vi "Add Custom Device to Sys Def.vi"(9 "Test Number":string="1", 10 "Custom Device Configuration File Path":path=path "C:/Users/admin/Desktop/Custom Device Tests/VeriStandProject/Custom Device Configurations/instrument_addon_udp_config.dat", 11 "nivssdfFile":string="C:\\Users\\admin\\Desktop\\Custom Device Tests\\VeriStandProject\\Instrument Custom Device Test.nivssdf") -> (0 "error out":errorcluster={"status"=TRUE, "code"=1430, "source"="Open/Create/Replace Datalog in Instrument System Definition API.lvlibp:Advanced System Definition.lvlib:Sysdef.LoadFile.vi->Instrument System Definition API.lvlibp:ImportExport.lvlib:File Interface.lvclass:Read File.vi->Instrument System Definition API.lvlibp:ImportExport.lvlib:Import Custom Device Configuration.vi->Instrument System Definition API.lvlibp:Create Instrument Custom Device.vi->Add Custom Device to Sys Def.vi<APPEND>\ninstrument_addon_udp_config.dat"}, 1 "SysDef Save error":string, 3 "Test Sys Def Path":string)   [LabVIEW 2015]
uses:
  Instrument System Definition API.lvlibp
  NationalInstruments.VeriStand.SystemDefinitionAPI
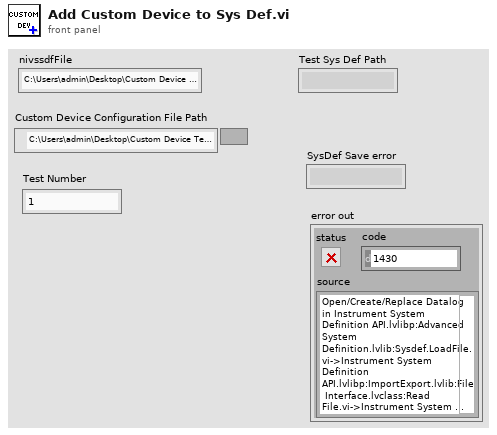
[diagram p1: front panel]
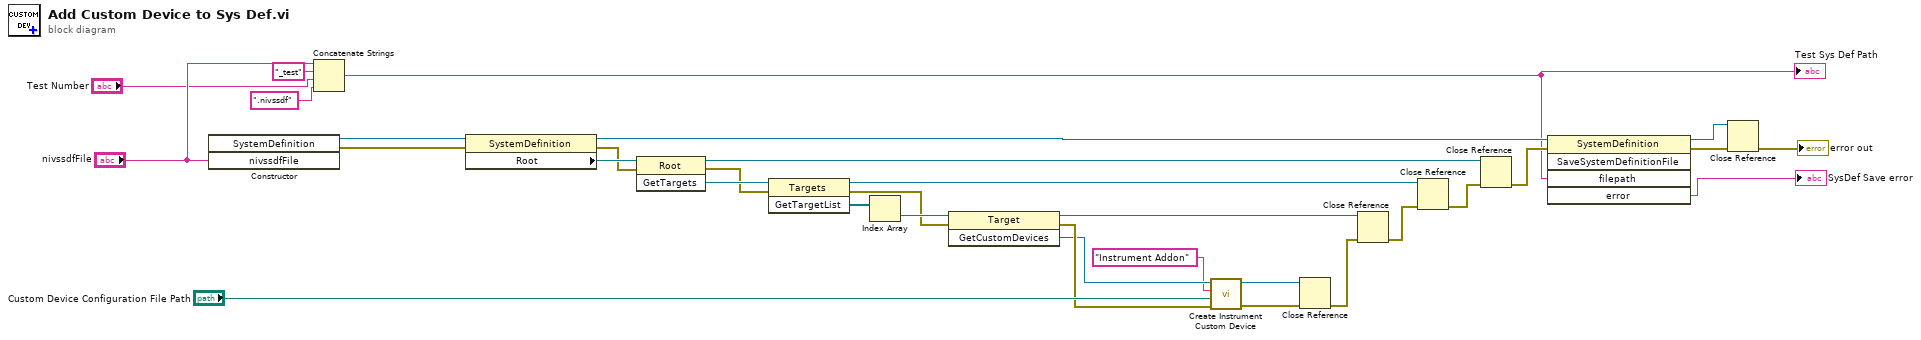
[diagram p0: block diagram]
diagram:
  n1 = constructor class="SystemDefinition"("nivssdfFile"="nivssdfFile") -> (reference out=w7:refnum<k24>, error out=w31:errorcluster)  [unwired: 3 in, 2 out]
  n2 = Concatenate Strings("nivssdfFile", "_test" ("string"), "Test Number", ".nivssdf" ("string")) -> (w3:string)
  "Test Sys Def Path" <- w3
  n3 = property class="SystemDefinition"(reference=w7, error in=w31) -> (reference out=w12:refnum<k24>, error out=w27:errorcluster, "Root"=w30:refnum<k24>)
  n4 = invoke class="Root" method="GetTargets"(reference=w30, error in=w27) -> (reference out=w14:refnum<k24>, error out=w28:errorcluster, "GetTargets"=w29:refnum<k24>)  [unwired: 1 in]
  n5 = invoke class="Targets" method="GetTargetList"(reference=w29, error in=w28) -> (reference out=w16:refnum<k24>, error out=w24:errorcluster, "GetTargetList"=w26:refnum<k24>[])  [unwired: 1 in]
  n6 = Index Array(array=w26) -> (element=w25:refnum<k24>)  [unwired: 1 in]
  n7 = invoke class="Target" method="GetCustomDevices"(reference=w25, error in=w24) -> (reference out=w18:refnum<k24>, error out=w23:errorcluster, "GetCustomDevices"=w22:refnum<k24>)  [unwired: 1 in]
  n8 = call "Create Instrument Custom Device.vi"("error in (no error)"=w23, "CD Config Path (.dat)"="Custom Device Configuration File Path", "Name"="Instrument Addon", "Custom Devices Ref"=w22) -> ("error out"=w19:errorcluster, "Custom Devices Ref"=w20:refnum<k24>)  [unwired: 6 in]
  n9 = Close Reference(reference=w20, error in (no error)=w19) -> (error out=w17:errorcluster)
  n10 = Close Reference(reference=w18, error in (no error)=w17) -> (error out=w15:errorcluster)
  n11 = Close Reference(reference=w16, error in (no error)=w15) -> (error out=w13:errorcluster)
  n12 = Close Reference(reference=w14, error in (no error)=w13) -> (error out=w11:errorcluster)
  n13 = invoke class="SystemDefinition" method="SaveSystemDefinitionFile"(reference=w12, error in=w11, "filepath"=w3) -> (reference out=w10:refnum<k24>, error out=w9:errorcluster, "error"=→"SysDef Save error":string)  [unwired: 2 in, 2 out]
  n14 = Close Reference(reference=w10, error in (no error)=w9) -> (error out=→"error out":errorcluster)
